vi "tkrsa6100 Config Frequency.vi"(0 "VISA Resource Name":refnum<visa-resource-name>, 5 "Set/Read\nFreq Setting (SET)":enum16{"SET", "READ"}(ring), 7 "Msmt Freq (MHz)\n(1000)":dbl=1000.0 min=0.009 max=20000.0 step=1e-06 format="%.6f", 11 "error in (no error)":errorcluster) -> (4 "dup VISA Resource Name":refnum<visa-resource-name>, 6 "Freq Setting\nResponse String":string, 15 "error out":errorcluster {"code" format="%#.0f"})   [LabVIEW 2020, in "Library Instrument & Equipement.lvlib" / "Library Spectrum Analyser.lvlib"]
doc: "Prerequisites for use:\n \nThis VI is valid in all measurement views.\n\nThis VI controls the following functions:\nThe frequency at which the current measurement will be run.\n\nerror in (no error) is checked by tkrsa6100 Write/Read wError Query.vi for any pending errors.\n\nIf error in status is ERROR:\n\nerror in (no error) and VISA Resource Name are passed straight through to error out and dup VISA Resource Name of the Write/Read Drivers and returned to the calling function. No commands are processed.\n\nIf error in status is NO ERROR:\n\nBy passing SET to Set/Read Freq Settings (SET) the measurement frequency can be written. Pass the desired frequency in MHz to numeric control Msmt Freq (MHz)(1000).\n\nOne command/query is executed per VI call.\n\nBy passing READ to enumerated control Set/Read Freq Settings (SET) the current measurement frequency can be queried. No other parameters necessary to be passed.\n\nValid return values are:\n\nRSA6106A 9KHz to 6GHz (in Hz)\nRSA6114A 9KHz to 14GHz (in Hz)\n\nThe appropriate command/query string is passed to tkrsa6100 Write/Read wError Query.vi. Input Error Query? is unwired so query SYST:ERR? is appended to the command string and any current error information is displayed in cluster Error Out.\n\nOn completion dup VISA Resource Name, Error Out, and Marker Setting Response String are returned to the calling function."
uses:
  Library Spectrum Analyser.lvlib
panel:
  # "RSA6100 Config Msmt Frequency Driver"
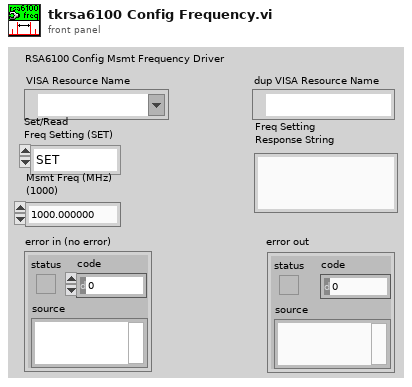
[diagram p1: front panel]
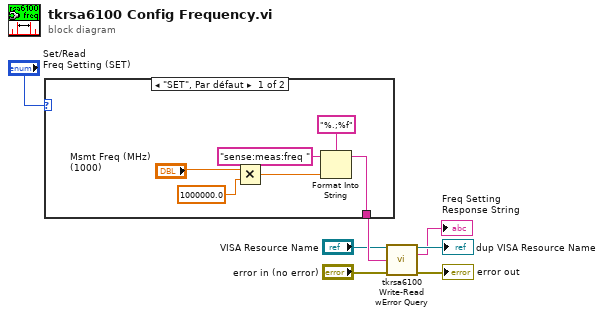
[diagram p0: block diagram]
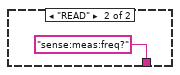
[diagram p2: hidden frame]
diagram:
  n1 = case shown="\"SET\", Par défaut" "Set/Read\nFreq Setting (SET)" {
    tunnel: [w9 "sense:meas:freq?" ("initial string")] -> w4
    frame "SET", Default {
      n2 = Multiply(x="Msmt Freq (MHz)\n(1000)", y=1000000.0) -> (x*y=w12:dbl)
      n3 = Format Into String(format string="%.;%f", initial string="sense:meas:freq ", w12) -> (resulting string=w9:string)  [unwired: 1 in, 1 out]
    }
    frame "READ" {
    }
  }
  n4 = call "tkrsa6100 Write-Read wError Query.vi"("VISA Resource Name"="VISA Resource Name", "Command (Empty String)"=w4, "error in (no error)"="error in (no error)") -> ("dup VISA Resource Name"=→"dup VISA Resource Name":refnum<visa-resource-name>, "Response"=→"Freq Setting\nResponse String":string, "error out"=→"error out":errorcluster)  [unwired: 4 in, 6 out]
